vi "Test(Dev)2Test(Data).vi"(8 "error in (no error)":errorcluster, 9 "log":string, 10 "Comment":string, 11 "TestInterface in":refnum<class "TestInterface.lvclass">) -> (0 "error out":errorcluster, 2 "DatenKlassen.lvlib:Test.lvclass out":refnum<class "Test.lvclass">, 3 "TestInterface out":refnum<class "TestInterface.lvclass">)   [LabVIEW 2013, in "EMV-Test.lvlib"]
uses:
  EMV-Test.lvlib
  classes/Datastructure/Test/Test.lvclass
  classes/Tests/TestInterface/TestInterface.lvclass
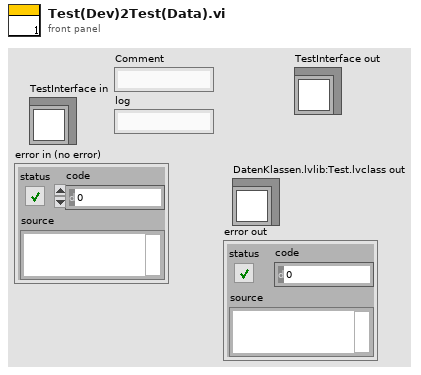
[diagram p1: front panel]
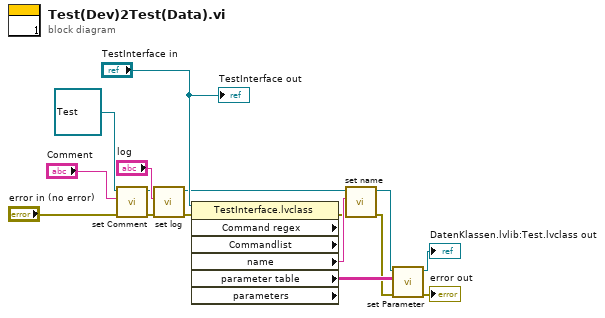
[diagram p0: block diagram]
diagram:
  n1 = call-dynamic "set Comment.vi"("error in (no error)"="error in (no error)", "Comment"="Comment", "Test (Eingang)"=refnum<class "Test.lvclass"> refnum ("DatenKlassen.lvlib:Test.lvclass 3")) -> ("error out"=w5:errorcluster, "Test (Ausgang)"=w2:refnum<class "Test.lvclass">)  [unwired: 7 in]
  n2 = call-dynamic "set log.vi"("error in (no error)"=w5, "log"="log", "Test (Eingang)"=w2) -> ("error out"=w4:errorcluster, "Test (Ausgang)"=w1:refnum<class "Test.lvclass">)  [unwired: 7 in]
  n3 = property class="TestInterface.lvclass" props=["Command regex", "Commandlist", "name", "parameter table", "parameters"](reference="TestInterface in", error in=w4) -> (error out=w12:errorcluster, "name"=w15:string, "parameter table"=w14:string[][])  [unwired: 4 out]
  n4 = call-dynamic "set name.vi"("error in (no error)"=w12, "name"=w15, "Test (Eingang)"=w1) -> ("error out"=w11:errorcluster, "Test (Ausgang)"=w13:refnum<class "Test.lvclass">)  [unwired: 7 in]
  n5 = call-dynamic "set Parameter.vi"("error in (no error)"=w11, "Parameter"=w14, "Test (Eingang)"=w13) -> ("error out"=→"error out":errorcluster, "Test (Ausgang)"=→"DatenKlassen.lvlib:Test.lvclass out":refnum<class "Test.lvclass">)  [unwired: 7 in]
  "TestInterface out" <- "TestInterface in"
